vi "Array-Masked Assignment.vi"(3 "Mask":bool[](array[boolean]), 4 "Value (NaN)":dbl=nan, 5 "Array In":dbl[](array[numeric])) -> (2 "Array Out":dbl[](array[numeric]))   [LabVIEW 2020]
doc: "Extracts the values from the input array for which the corresponding boolean inputs are TRUE."
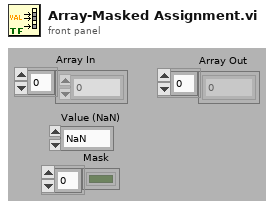
[diagram p1: front panel]
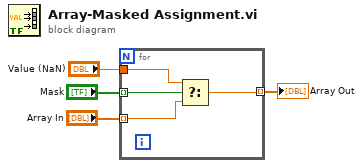
[diagram p0: block diagram]
diagram:
  n1 = for {
    tunnel: "Mask" -> [w8] mode=indexing
    tunnel: "Array In" -> [w7] mode=indexing
    tunnel: [w6] -> w2 mode=indexing
    tunnel: "Value (NaN)" -> [w5]
    n2 = Select(t=w5, s=w8, f=w7) -> (s? t:f=w6:dbl)
  }
  "Array Out" <- w2
